vi "Update SubPanel.vi"(8 "error in (no error)":errorcluster, 11 "Manager in":refnum<class "Manager.lvclass">) -> (0 "error out":errorcluster, 3 "Manager out":refnum<class "Manager.lvclass">)   [LabVIEW 2013, in "Manager.lvlib" / "Manager.lvclass"]
uses:
  Manager.lvclass
  Manager.lvclass/Manager.ctl
  Read Control Systems.vi
  Read System Ring Refnum.vi
  Read Actor Ring Refnum.vi
  Read SubPnl Refnum.vi
  PluginInterface/Actor Framework.lvlibp/Message Enqueuer/Message Enqueuer.lvclass
  PluginInterface/PluginInterface.lvlibp/PluginInterfaceClass/View Front Panel Msg.lvclass
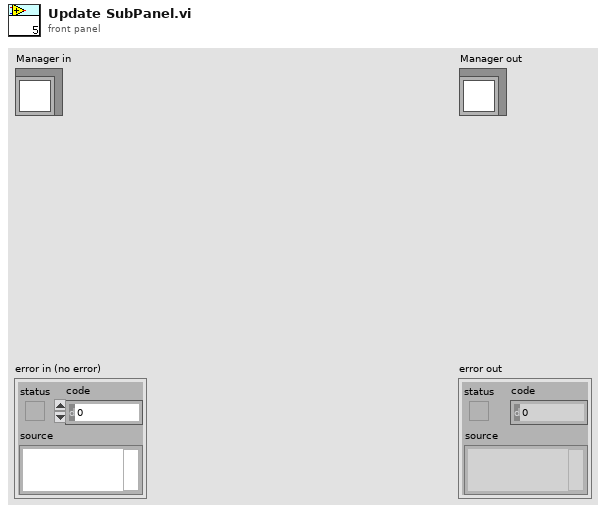
[diagram p1: front panel]
types:
  T1 = cluster{"Name":string, "Plugins":refnum<class "Message Enqueuer.lvclass">[]}[]
  T2 = cluster{"Name":string, "Plugins":refnum<class "Message Enqueuer.lvclass">[]}
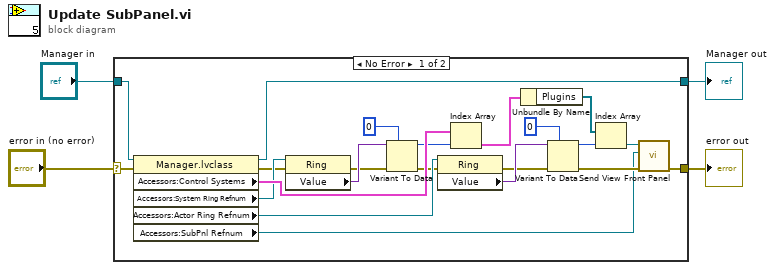
[diagram p0: block diagram]
diagram:
  n1 = case shown="No Error" "error in (no error)" {
    selector: "error in (no error)" -> [w15 w28]
    tunnel: [w7 w28] -> w3
    tunnel: [w16 w27] -> w1
    tunnel: "Manager in" -> [w26 w27]
    frame No Error {
      n2 = property class="Manager.lvclass"(reference=w26, error in=w15) -> (reference out=w16:refnum<class "Manager.lvclass">, error out=w14:errorcluster, "Accessors:Control Systems"=w25:T1, "Accessors:System Ring Refnum"=w24:refnum<vi>, "Accessors:Actor Ring Refnum"=w18:refnum<vi>, "Accessors:SubPnl Refnum"=w6:refnum<vi>)
      n3 = property class="Ring"(reference=w24, error in=w14) -> (error out=w13:errorcluster, "Value"=w22:variant)  [unwired: 1 out]
      n4 = Variant To Data(error in=w13, type=0, Variant=w22) -> (data=w21:i32, error out=w12:errorcluster)
      n5 = property class="Ring"(reference=w18, error in=w12) -> (error out=w11:errorcluster, "Value"=w19:variant)  [unwired: 1 out]
      n6 = Index Array(array=w25, index=w21) -> (element=w17:T2)
      n7 = Unbundle By Name(w17) -> ("Plugins"=w10:refnum<class "Message Enqueuer.lvclass">[])
      n8 = Variant To Data(error in=w11, type=0, Variant=w19) -> (data=w9:i32, error out=w8:errorcluster)
      n9 = Index Array(array=w10, index=w9) -> (element=w5:refnum<class "Message Enqueuer.lvclass">)
      n10 = call "Send View Front Panel.vi"("error in (no error)"=w8, "SubPnl Refnum"=w6, "Message Enqueuer"=w5) -> ("error out"=w7:errorcluster)  [unwired: 7 in, 1 out]
    }
    frame Error {
    }
  }
  "error out" <- w3
  "Manager out" <- w1
